vi "Process.vi"(8 "error in":errorcluster, 11 "Inst UI.AH2500":refnum<class "Inst UI.AH2500.lvclass">) -> (0 "error out":errorcluster, 3 "Inst UI.AH2500 out":refnum<class "Inst UI.AH2500.lvclass">)   [LabVIEW 2019, in "Inst UI.AH2500.lvclass"]
doc: "---------------------------------------------------------------\nJKI State Machine Objects™\nhttp://jki.net/state-machine-objects/\nCopyright (C) 2005-2015, JKI <info@jki.net>\nALL RIGHTS RESERVEDJKI State Machine Objects (SMO) 1.0.0.5\nJKI - JKI\nCopyright (c) 2016, JKI"
uses:
  Inst UI.AH2500.lvclass
  C:/Program Files/National Instruments/LabVIEW 2019/vi.lib/JKI/JKI SMO/SMO/SMO.lvclass
  C:/Program Files/National Instruments/LabVIEW 2019/user.lib/LevyLab/Instrument Framework/Instrument UI/Instrument UI.lvclass
  C:/Program Files/National Instruments/LabVIEW 2019/vi.lib/JKI/JKI SMO/SMO.UI/SMO.UI.lvclass
  Inst.AH2500/Typedefs/Inst.AH2500.getAll--Cluster.ctl
  Inst.AH2500/Inst.AH2500.lvclass
  C:/Program Files/National Instruments/LabVIEW 2019/user.lib/LevyLab/Instrument Framework/Instrument/Instrument.lvclass
  Inst UI.AH2500.UI--Cluster.ctl
  Inst.AH2500/Typedefs/Inst.AH2500.Configuration--Cluster.ctl
  <userlib>/LevyLab/Configuration/Configuration.lvclass
  <userlib>/LevyLab/RemoteControl/RemoteControl/Typedefs/Message--Cluster.ctl
  <userlib>/LevyLab/Instrument Framework/Instrument UI/Instrument UI.lvclass/Instrument UI.ctl
  Inst.AH2500/Inst.AH2500.lvclass/Inst.AH2500.ctl
  <vilib>/JKI/JKI SMO/SMO/SMO.lvclass/SMO.ctl
  <userlib>/LevyLab/Configuration/Configuration.lvclass/Configuration.ctl
  <userlib>/LevyLab/Instrument Framework/Instrument/Typedefs/Client Type--Enum.ctl
  <userlib>/LevyLab/Instrument Framework/Instrument/Instrument.lvclass/Instrument.ctl
  f57a6be4-1a14-4c07-88ea-2903807e6527.vi
  <vilib>/JKI/JKI SMO/SMO/Private/ReftoDVR--SMO.vi
  f57a6be4-1a14-4c07-88ea-2903807e6527.vi/3b87bc3d-4873-4b4f-ba08-c078dcd240b2.vi
  f57a6be4-1a14-4c07-88ea-2903807e6527.vi/f27b08c5-9c53-421b-9d46-0768e3ef8b01.vi
  <vilib>/Utility/Data Type/Get Type Information.vi
  <vilib>/JDP Science/JSONtext/JSON text to Variant.vi
  <userlib>/LevyLab/Instrument Framework/Instrument/API/Instrument.sendMessageToProcess (variant).vi
  <userlib>/LevyLab/Instrument Framework/Instrument/Instrument.lvclass
  <vilib>/JDP Science/JSONtext/LVClass Serializer/JSONtext LVClass Serializer.lvclass
  <userlib>/LevyLab/Instrument Framework/Instrument UI/Instrument UI.lvclass
  <vilib>/JKI/JKI SMO/SMO/SMO.lvclass
  <vilib>/JKI/JKI SMO/SMO.UI/SMO.UI.lvclass
  <userlib>/LevyLab/RemoteControl/RemoteControl/RemoteControl.lvclass
  C:/Program Files/National Instruments/LabVIEW 2019/user.lib/LevyLab/Instrument Framework/Instrument Types/CBridge/Instrument.CBridge.lvclass
panel:
  in  "Enable Output 2":bool
  in  "I/O":bool
  out "STUFF":bool
  out "LOSS":string="bridge"
  out "CAPACITANCE - pF":string="cap"
  out "Status":string="SMO State: Stopped"
  out "version":string="vDevelopment"
  # "AH 2500A ULTRA-PRECISION 1kHz CAPACITANCE BRIDGE"
  # "SMO UI Template"
  # "For instructions on how to use the JKI State Machine Objects, examples and video tutorials, visit:\nhttp://jki.net/state-machine-objects/\n\nJKI State Machine Objects™\nhttp://jki.net/state-machine-objects/\nCopyright (C) 2005-2015, JKI <info@jki.net>\nALL RIGHTS RESERVED"
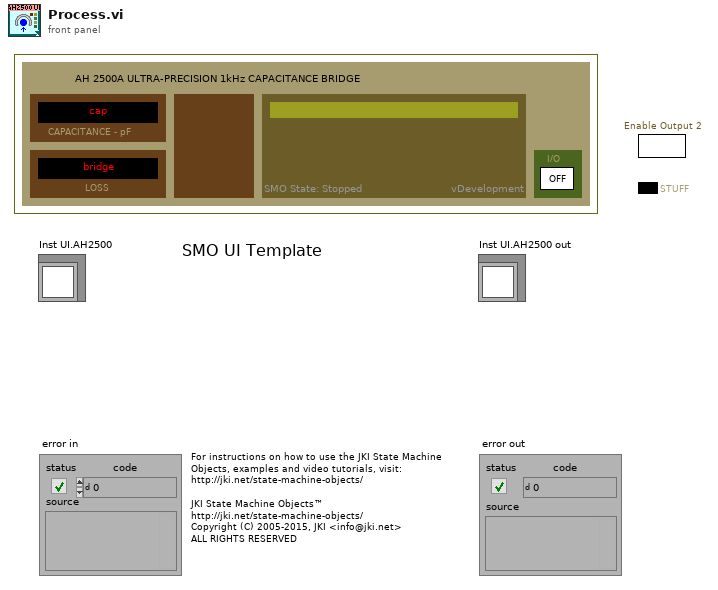
[diagram p1: front panel]
types:
  T1 = enum32{"invalid app kind", "Development System", "Run Time System", "Student Edition", "Embedded LabVIEW", "Evaluation", "Custom"}
  T2 = enum32{"Invalid", "Standard", "Closed", "Hidden", "Minimized", "Maximized"}
  T3 = typedef "Instrument.lvlib/Instrument.lvclass/Client Type--Enum.ctl" = enum16{"Remote", "Local"}
  T4 = typedef "RemoteControl.lvclass/Message--Cluster.ctl" = cluster{"Command":string, "Data":variant, "ID":string}
  T5 = typedef "Inst.AH2500.lvclass/Inst.AH2500.Configuration--Cluster.ctl" = cluster{"Example Setting 1":dbl, "Example Setting 2":dbl, "Example Setting 3":string}
  T6 = typedef "Inst.AH2500.lvclass/Inst.AH2500.getAll--Cluster.ctl" = cluster{"capacitance (pF)":dbl, "loss (nS)":dbl, "Vexc (V)":dbl}
  T7 = typedef "Inst UI.AH2500.lvclass/Inst UI.AH2500.UI--Cluster.ctl" = cluster{"Ch1 (V)":dbl, "Ch2 (V)":dbl, "Slew (V/s)":dbl}
  T8 = typedef "RemoteControl.lvlib/RemoteControl.lvclass/Message--Cluster.ctl" = cluster{"Command":string, "Data":variant, "ID":string}
  T9 = cluster{"Core":cluster{"Current VI Reference":refnum<vi>, "Close Panel on Exit?":bool, "Last Error":cluster{"error":errorcluster, "previous state":string, "remaining states":string}, "Shutdown?":bool}, "Instrument UI":refnum<class "Inst UI.AH2500.lvclass">, "Instrument":refnum<class "Inst.AH2500.lvclass">, "Configuration":refnum<class "Configuration.lvclass">, "Config Cluster":T5, "getAll":T6, "UI Cluster":T7, "Message":T8}
  T10 = cluster{"Current VI Reference":refnum<vi>, "Close Panel on Exit?":bool, "Last Error":cluster{"error":errorcluster, "previous state":string, "remaining states":string}, "Shutdown?":bool}
  T11 = typedef "SMO.lvclass/SMOState --Enum.ctl" = enum16{"unknown", "Created", "Started", "Stopped"}
  T12 = typedef "SMO.lvclass/Protected Events.ctl" = cluster{"StopProcesses":refnum<user-event>, "AbortProcesses":refnum<user-event>, "Config Changed":refnum<user-event>, "Dependency":refnum<user-event>}
  T13 = typedef "Instrument.lvlib/Instrument.lvclass/PublicEvents--Cluster.ctl" = cluster{"MessageFromProcess":refnum<user-event>}
  T14 = typedef "Inst.AH2500.lvclass/PublicEvents--Cluster.ctl" = cluster{"MessageFromProcess":refnum<user-event>}
  T15 = typedef "SMO.lvclass/Public Events.ctl" = cluster{"Error":refnum<user-event>, "State":refnum<user-event>, "Reserve State":refnum<user-event>}
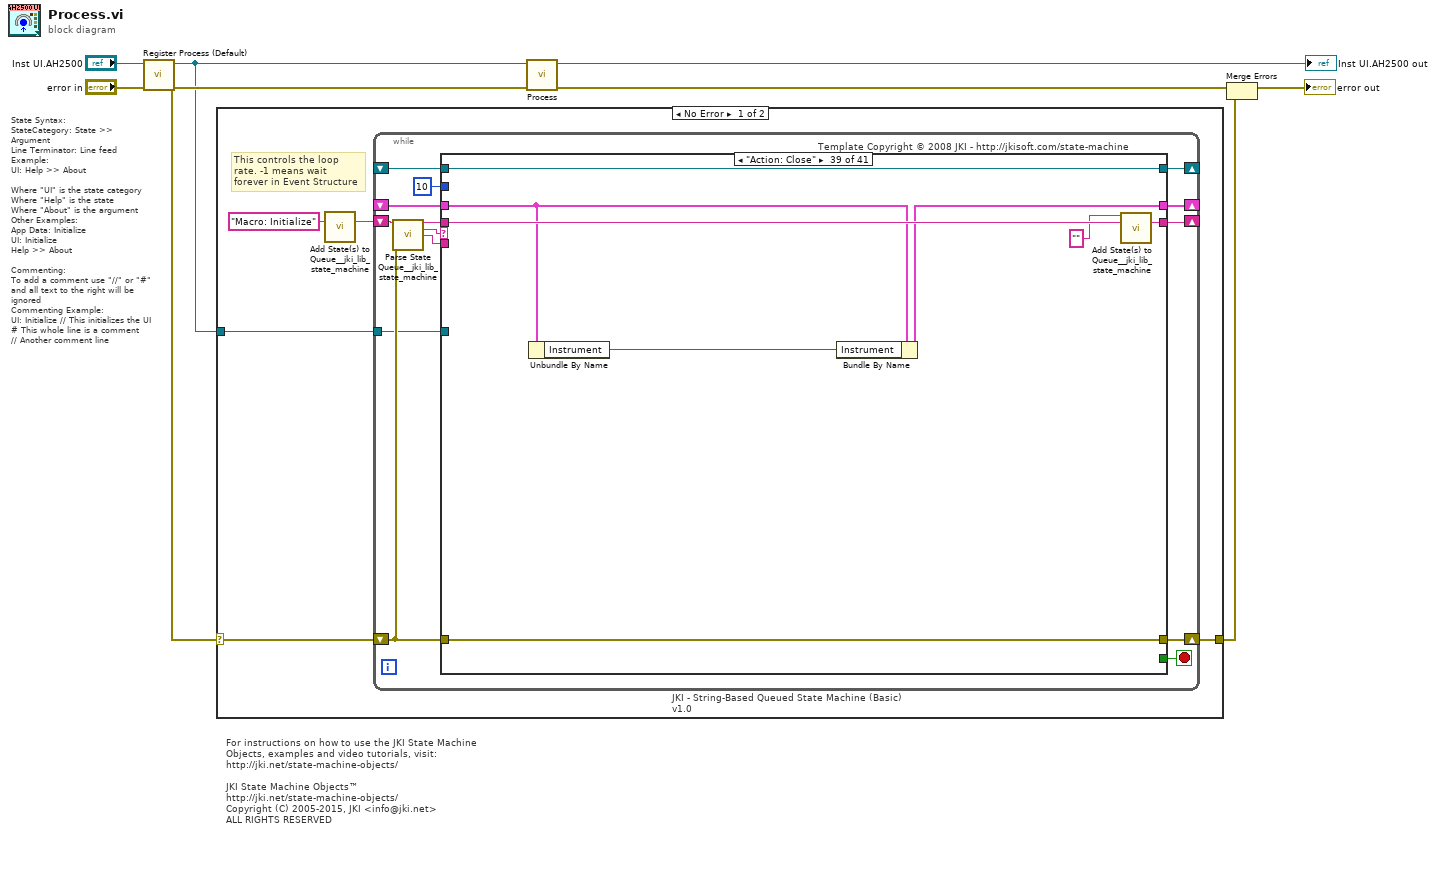
[diagram p0: block diagram]
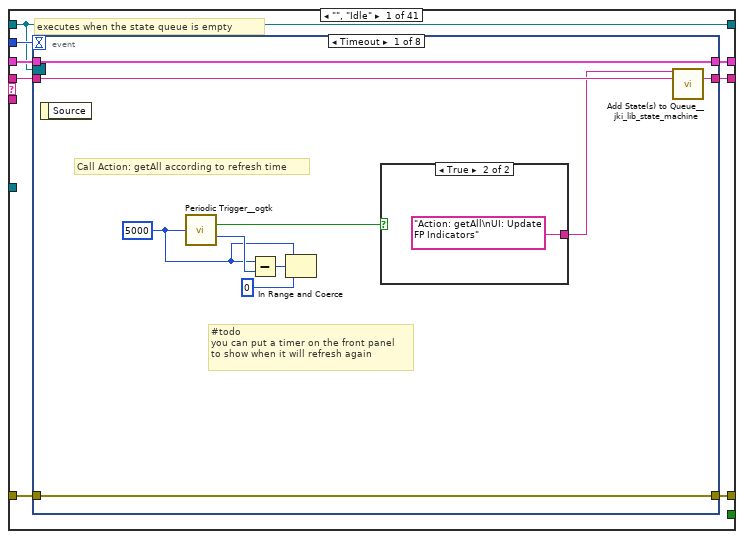
[diagram p2: hidden frame]
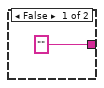
[diagram p3: hidden frame]
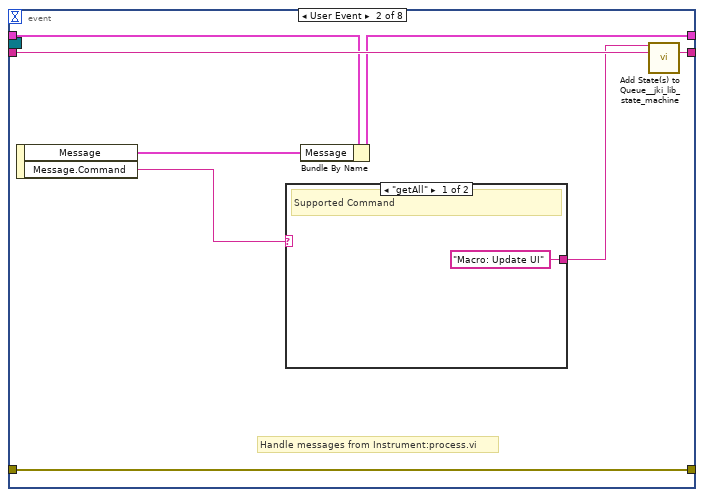
[diagram p4: hidden frame]
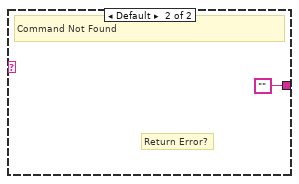
[diagram p5: hidden frame]
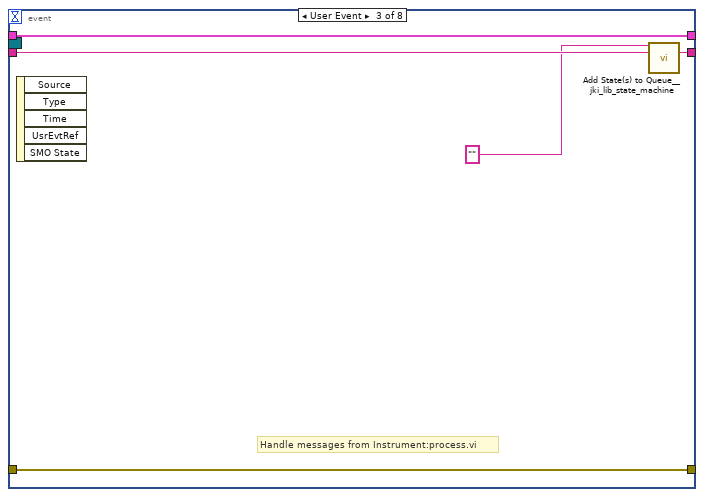
[diagram p6: hidden frame]
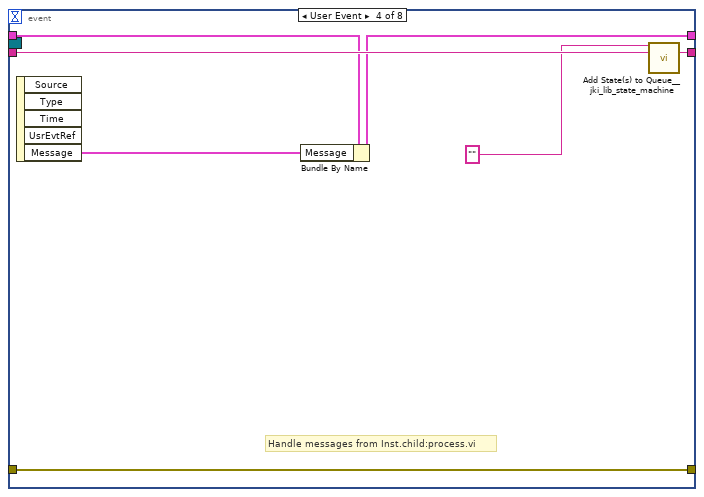
[diagram p7: hidden frame]
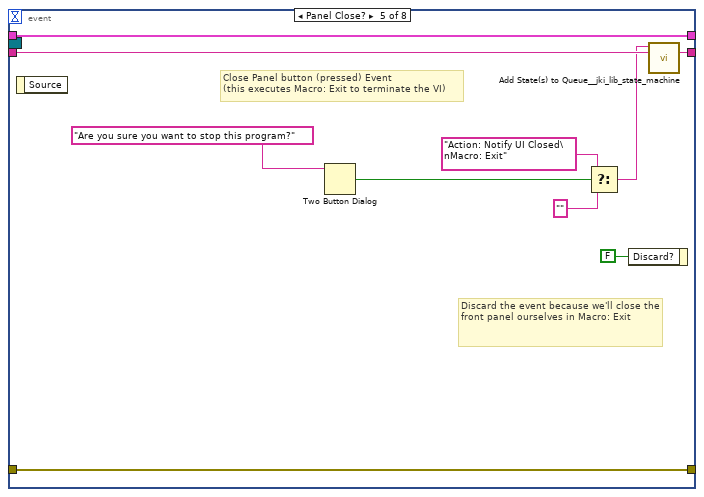
[diagram p8: hidden frame]
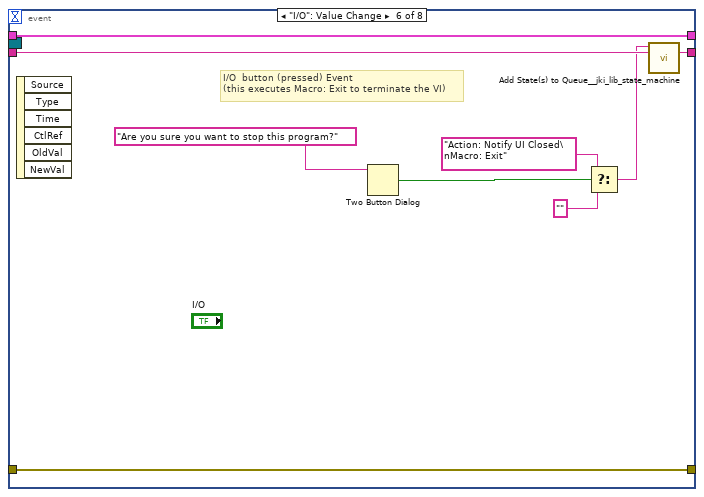
[diagram p9: hidden frame]
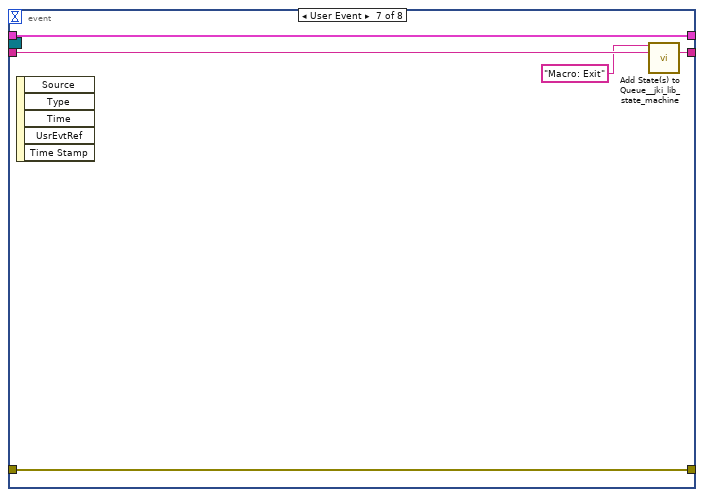
[diagram p10: hidden frame]
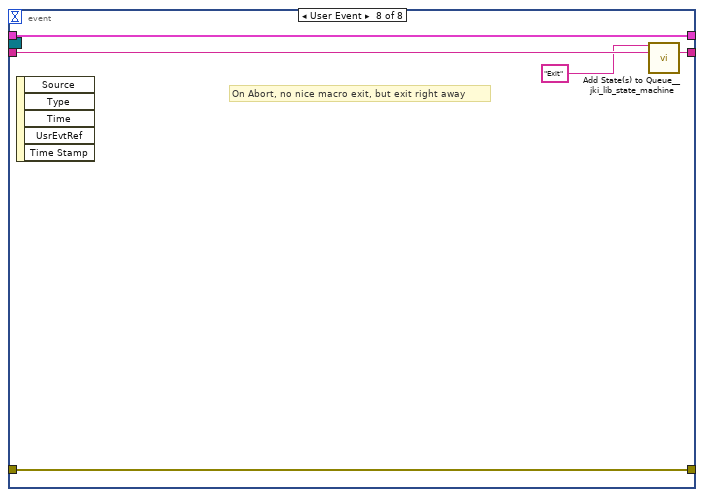
[diagram p11: hidden frame]
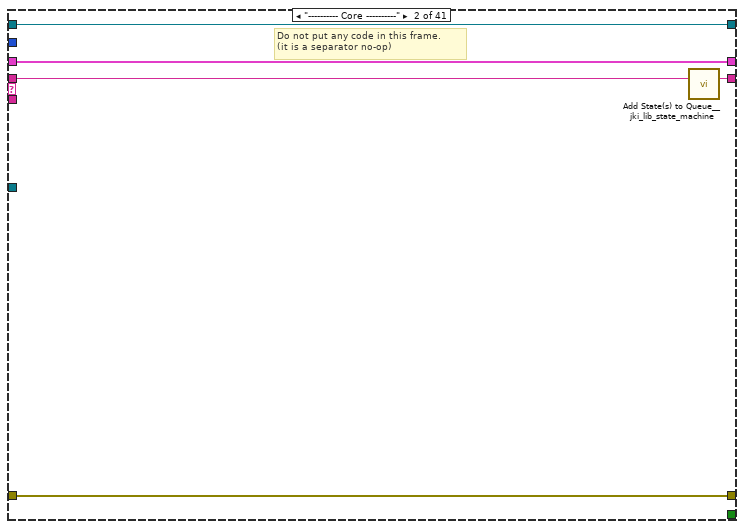
[diagram p12: hidden frame]
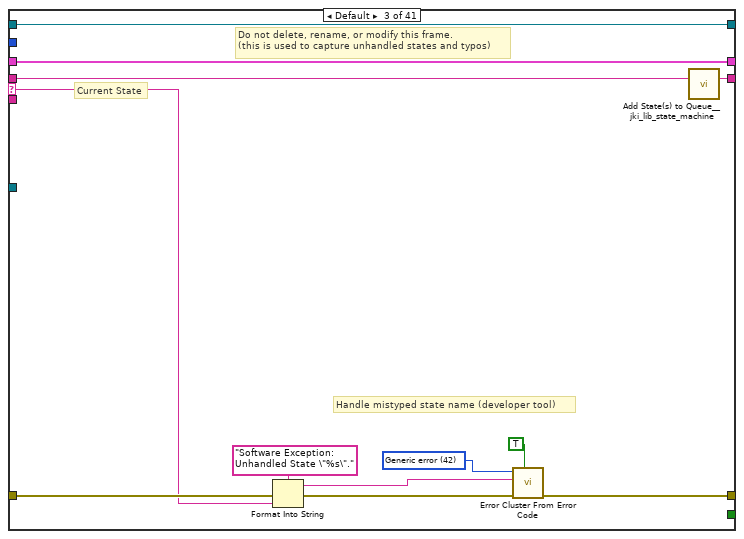
[diagram p13: hidden frame]
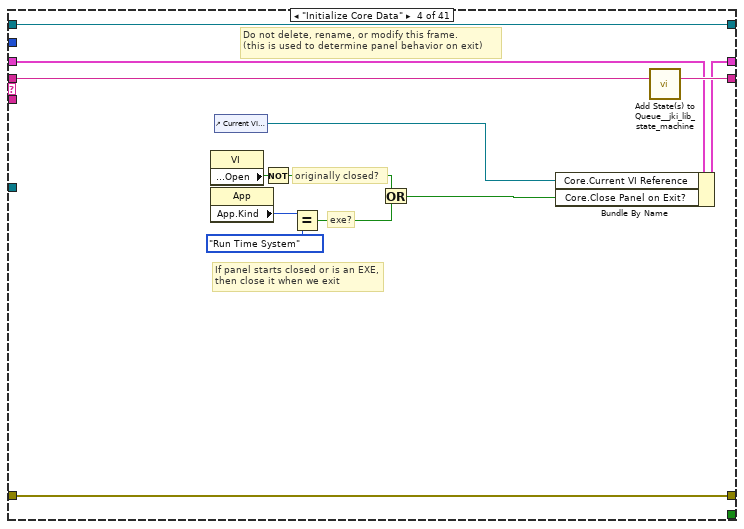
[diagram p14: hidden frame]
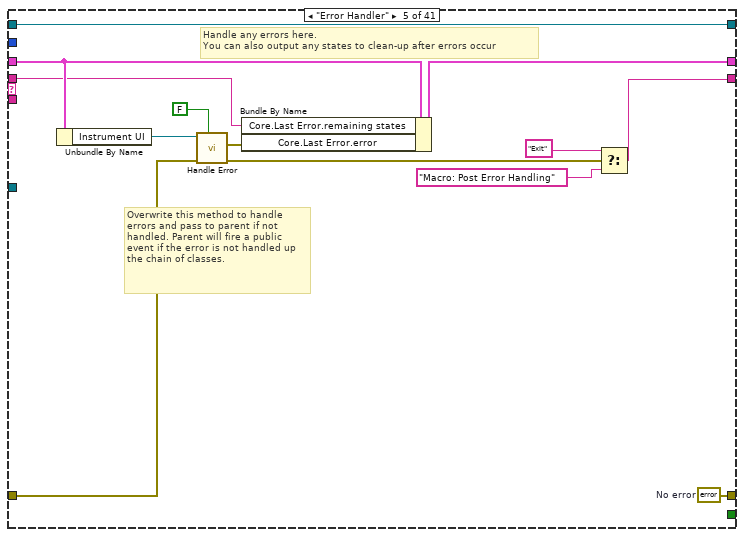
[diagram p15: hidden frame]
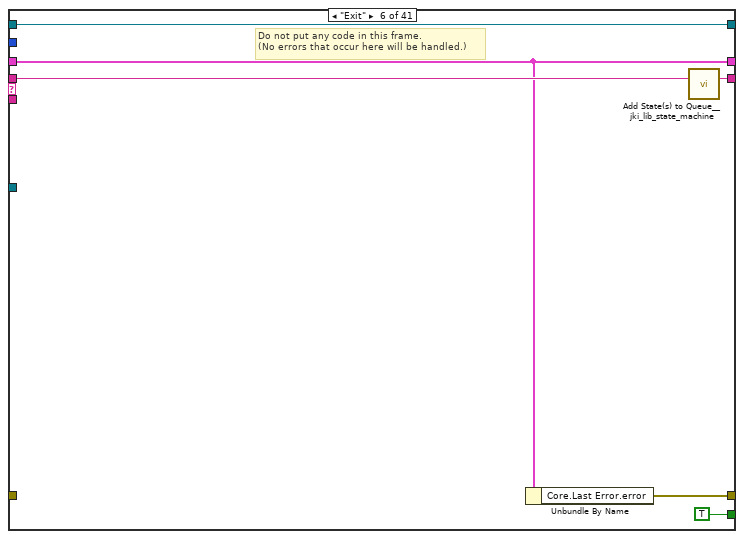
[diagram p16: hidden frame]
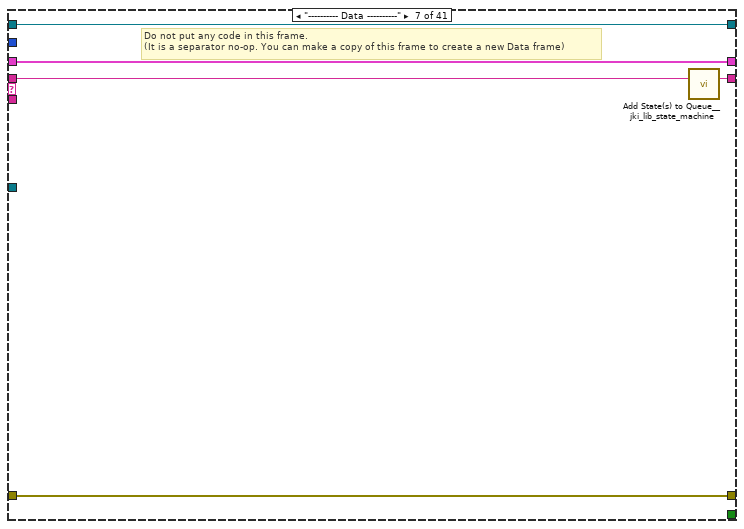
[diagram p17: hidden frame]
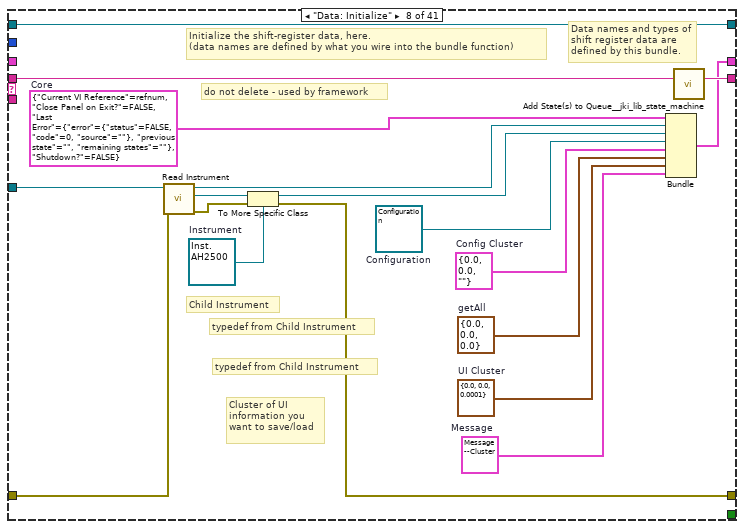
[diagram p18: hidden frame]
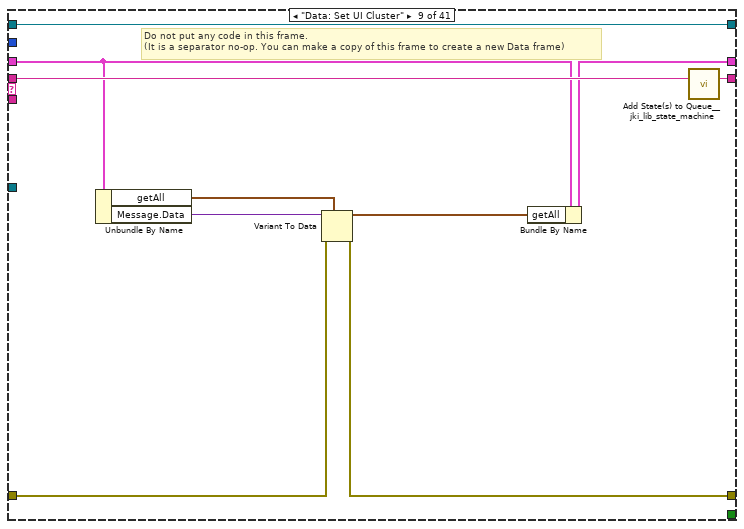
[diagram p19: hidden frame]
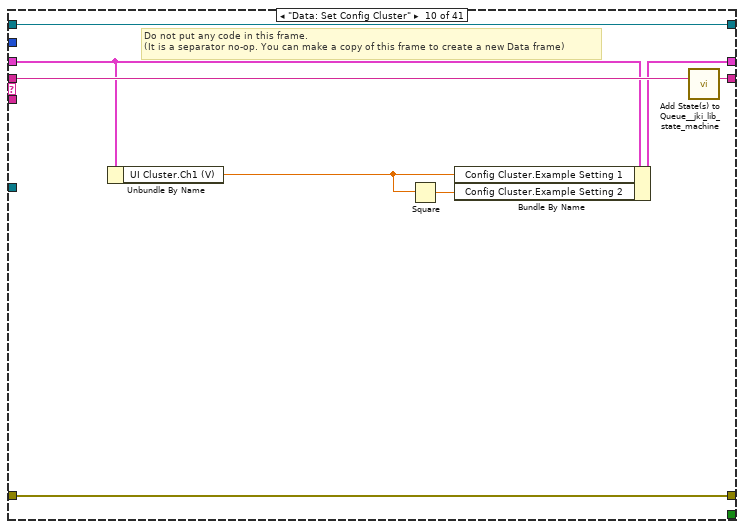
[diagram p20: hidden frame]
diagram:
  # "State Syntax:\nStateCategory: State >> Argument\nLine Terminator: Line feed\nExample:\nUI: Help >> About\n\nWhere \"UI\" is the state category\nWhere \"Help\" is the state\nWhere \"About\" is the argument\nOther Examples:\nApp Data: Initialize\nUI: Initialize\nHelp >> About\n\nCommenting:\nTo add a comment use \"//\" or \"#\" and all text to the right will be ignored\nCommenting Example:\nUI: Initialize // This initializes the UI\n# This whole line is a comment\n// Another comment line"
  # "For instructions on how to use the JKI State Machine Objects, examples and video tutorials, visit:\nhttp://jki.net/state-machine-objects/\n\nJKI State Machine Objects™\nhttp://jki.net/state-machine-objects/\nCopyright (C) 2005-2015, JKI <info@jki.net>\nALL RIGHTS RESERVED"
  n1 = call <vilib>:"Register Process (Default).vi"("error in (no error)"="error in", "SMO"="Inst UI.AH2500") -> ("error out"=w5:errorcluster, "SelfRef"=w4:refnum<class "Inst UI.AH2500.lvclass">)  [unwired: 8 in]
  n2 = case shown="No Error" w5 {
    selector: w5 -> [w10 w509]
    tunnel: w4 -> [w11 _]
    tunnel: [w9 w509] -> w1
    frame No Error {
      # "This controls the loop rate. -1 means wait forever in Event Structure"
      n3 = call <vilib>:"Add State(s) to Queue__jki_lib_state_machine.vi"("State(s) in (\"\")"="Macro: Initialize") -> ("States Out"=w13:string)  [unwired: 14 in]
      n4 = while "JKI - String-Based Queued State Machine (Basic) v1.0" {
        shift-right: [w20] -> _
        shift-left: _ -> [w19]
        shift-right: [w23] -> w9
        shift-left: w10 -> [w17]
        shift-right: [w22] -> _
        shift-left: w13 -> [w24]
        tunnel: w11 -> [w16]
        shift-right: [w15] -> _
        shift-left: _ -> [w14]
        stop <- w21 stop-if-true
        # "Template Copyright © 2008 JKI - http://jkisoft.com/state-machine"
        n5 = call <vilib>:"Parse State Queue__jki_lib_state_machine.vi"("State Queue"=w24, "Error In (no error)"=w17) -> ("Remaining States"=w26:string, "Current State"=w27:string, "Arguments"=w25:string)  [unwired: 11 in]
        n6 = case shown="\"Action: Close\"" w27 {
          selector: w27 -> [_ _ w105 _ _ _ _ _ _ _ _ _ _ _ _ _ _ _ _ _ _ _ _ _ _ _ _ _ _ _ _ _ _ _ _ _ _ _ _ _ _]
          tunnel: w26 -> [w35 w103 w109 w128 w132 w147 w152 w170 w180 w188 w195 w200 w212 w217 w231 w242 w258 w290 w299 w311 w321 w327 w333 w348 w353 w364 w371 w376 w395 w401 w406 w421 w429 w441 w448 w455 w469 w480 w488 w498 w508]
          tunnel: w25 -> [_ _ _ _ _ _ _ _ _ _ _ _ _ _ _ w236 w252 _ _ _ _ _ _ _ _ _ _ _ _ _ _ _ _ _ _ _ _ _ _ _ _]
          tunnel: w19 -> [w33 w100 w107 w119 w135 w143 w149 _ w176 w184 w189 w197 w210 w213 w227 w240 w254 w287 w295 w301 w318 w324 w330 w335 w350 w361 w366 w373 w393 w399 w403 w414 w426 w432 w443 w449 w462 w475 w481 w493 w503]
          tunnel: [w32 w101 w111 w125 w137 w142 w150 w157 w172 w186 w191 w198 w207 w215 w228 w237 w255 w288 w297 w309 w319 w325 w331 w346 w351 w355 w367 w374 w390 w396 w404 w407 w424 w433 w445 w450 w457 w472 w482 w489 w499] -> w23
          tunnel: w17 -> [w31 w101 w110 w125 w131 _ w150 w154 w171 w186 w192 w198 w208 w215 w228 w238 w256 w288 w297 w309 w319 w325 w331 w346 w351 w356 w368 w374 w380 w397 w404 w416 w422 w434 w445 w451 w463 w471 w482 w490 w500]
          tunnel: [w34 w102 w108 w127 w129 w146 w151 w169 w179 w187 w194 w199 w211 w216 w230 w241 w257 w289 w298 w310 w320 w326 w332 w347 w352 w363 w370 w375 w394 w400 w405 w420 w428 w440 w447 w454 w468 w479 w487 w497 w507] -> w22
          tunnel: [_ _ _ _ _ TRUE _ _ _ _ _ _ _ _ _ _ _ _ _ _ _ _ _ _ _ _ _ _ _ _ _ _ _ _ _ _ _ _ _ _ _] -> w21
          tunnel: [w30 w100 w107 w126 w134 w143 w149 w168 w177 w183 w189 w197 w210 w213 w227 w240 w254 w287 w295 w302 w318 w324 w330 w335 w350 w361 w366 w373 w393 w399 w403 w418 w426 w430 w442 w449 w464 w476 w483 w494 w504] -> w20
          tunnel: 10 ("Timeout") -> [w29 _ _ _ _ _ _ _ _ _ _ _ _ _ _ _ _ _ _ _ _ _ _ _ _ _ _ _ _ _ _ _ _ _ _ _ _ _ _ _ _]
          tunnel: w16 -> [_ _ _ _ _ _ _ w155 _ _ _ _ _ _ _ _ _ _ _ _ _ _ _ _ _ _ _ _ _ _ _ _ _ _ _ _ _ _ _ _ _]
          tunnel: [w28 w99 w104 w116 w141 w144 w148 w167 w178 w185 w190 w196 w209 w214 w229 w239 w251 w286 w296 w308 w317 w323 w329 w340 w349 w362 w369 w372 w392 w398 w402 w419 w427 w439 w446 w453 w467 w478 w486 w496 w506] -> w15
          tunnel: w14 -> [w28 w99 w104 w116 w141 w144 w148 w167 w178 w185 w190 w196 w209 w214 w229 w239 w251 w286 w296 w308 w317 w323 w329 w340 w349 w362 w369 w372 _ w398 w402 w419 w427 w439 w446 w453 w467 w478 w486 w496 w506]
          frame "", "Idle" {
            # "executes when the state queue is empty"
            n7 = event shown="[0] Timeout" {
              selector: w28 -> [_ _ _ _ _ _ _ _]
              dyn-events: _ -> [_ _ _ _ _ _ _ _]
              timeout: w29 -> [_ _ _ _ _ _ _ _]
              tunnel: w35 -> [w45 w55 w62 w69 w79 w88 w93 w98]
              tunnel: [w44 w54 w61 w68 w78 w87 w92 w97] -> w34
              tunnel: w33 -> [w42 w52 w58 w66 w76 w86 w90 w95]
              tunnel: [w43 w53 w60 w67 w75 w85 w91 w96] -> w32
              tunnel: w31 -> [w43 w53 w60 w67 w75 w85 w91 w96]
              tunnel: [w42 w51 w58 w65 w76 w86 w90 w95] -> w30
              event Timeout {
                w37 = u32 5000 ("time (ms)")
                # "#todo\nyou can put a timer on the front panel\nto show when it will refresh again"
                # "Call Action: getAll according to refresh time"
                n8 = event-data() -> ()  [unwired: 1 in, 1 out]
                n9 = call <userlib>:"Periodic Trigger__ogtk.vi"("time (ms)"=w37) -> ("Triggered"=w40:bool, "timer value"=w39:u32)  [unwired: 12 in, 1 out]
                n10 = Subtract(x=w37, y=w39) -> (x-y=w38:u32)
                n11 = In Range and Coerce(upper limit=w37, x=w38, lower limit=u32 0) -> ()  [unwired: 2 out]
                n12 = case shown="True" w40 {
                  tunnel: ["" ("State(s) in Front (\"\")") "Action: getAll\nUI: Update FP Indicators" ("State(s) in Front (\"\")")] -> w41
                  frame False {
                  }
                  frame True {
                  }
                }
                n13 = call <vilib>:"Add State(s) to Queue__jki_lib_state_machine.vi"("State(s) in Front (\"\")"=w41, "State(s) in (\"\")"=w45) -> ("States Out"=w44:string)  [unwired: 13 in]
              }
              event User Event {
                # "Handle messages from Instrument:process.vi"
                n14 = event-data() -> ("Message"=w50:T4, "Message.Command"=w48:string)  [unwired: 1 in]
                n15 = case shown="\"getAll\"" w48 {
                  tunnel: ["Macro: Update UI" "" ("Empty String Constant")] -> w49
                  frame "getAll" {
                    # "Supported Command"
                  }
                  frame Default {
                    # "Return Error?"
                    # "Command Not Found"
                  }
                }
                n16 = Bundle By Name(cluster=w52, "Message"=w50) -> (w51:T9)
                n17 = call <vilib>:"Add State(s) to Queue__jki_lib_state_machine.vi"("State(s) in Front (\"\")"=w49, "State(s) in (\"\")"=w55) -> ("States Out"=w54:string)  [unwired: 13 in]
              }
              event User Event {
                # "Handle messages from Instrument:process.vi"
                n18 = event-data() -> ()  [unwired: 1 in, 5 out]
                n19 = call <vilib>:"Add State(s) to Queue__jki_lib_state_machine.vi"("State(s) in Front (\"\")"="" ("State(s) in Front (\"\")"), "State(s) in (\"\")"=w62) -> ("States Out"=w61:string)  [unwired: 13 in]
              }
              event User Event {
                # "Handle messages from Inst.child:process.vi"
                n20 = event-data() -> ("Message"=w63:T4)  [unwired: 1 in, 4 out]
                n21 = Bundle By Name(cluster=w66, "Message"=w63) -> (w65:T9)
                n22 = call <vilib>:"Add State(s) to Queue__jki_lib_state_machine.vi"("State(s) in Front (\"\")"="" ("State(s) in Front (\"\")"), "State(s) in (\"\")"=w69) -> ("States Out"=w68:string)  [unwired: 13 in]
              }
              event Panel Close? {
                # "Discard the event because we'll close the front panel ourselves in Macro: Exit"
                # "Close Panel button (pressed) Event\n(this executes Macro: Exit to terminate the VI)"
                n23 = event-data() -> ()  [unwired: 1 in, 1 out]
                n24 = Two Button Dialog(message="Are you sure you want to stop this program?") -> (T button?=w74:bool)  [unwired: 2 in]
                n25 = Select(t="Action: Notify UI Closed\nMacro: Exit", s=w74, f="") -> (s? t:f=w71:string)
                n26 = event-data("Discard?"=FALSE) -> ()  [unwired: 1 in, 1 out]
                n27 = call <vilib>:"Add State(s) to Queue__jki_lib_state_machine.vi"("State(s) in Front (\"\")"=w71, "State(s) in (\"\")"=w79) -> ("States Out"=w78:string)  [unwired: 13 in]
              }
              event "I/O": Value Change {
                # "I/O  button (pressed) Event\n(this executes Macro: Exit to terminate the VI)"
                n28 = event-data() -> ()  [unwired: 1 in, 6 out]
                n29 = Two Button Dialog(message="Are you sure you want to stop this program?") -> (T button?=w84:bool)  [unwired: 2 in]
                n30 = Select(t="Action: Notify UI Closed\nMacro: Exit", s=w84, f="") -> (s? t:f=w81:string)
                n31 = call <vilib>:"Add State(s) to Queue__jki_lib_state_machine.vi"("State(s) in Front (\"\")"=w81, "State(s) in (\"\")"=w88) -> ("States Out"=w87:string)  [unwired: 13 in]
              }
              event User Event {
                n32 = event-data() -> ()  [unwired: 1 in, 5 out]
                n33 = call <vilib>:"Add State(s) to Queue__jki_lib_state_machine.vi"("State(s) in Front (\"\")"="Macro: Exit", "State(s) in (\"\")"=w93) -> ("States Out"=w92:string)  [unwired: 13 in]
              }
              event User Event {
                # "On Abort, no nice macro exit, but exit right away"
                n34 = event-data() -> ()  [unwired: 1 in, 5 out]
                n35 = call <vilib>:"Add State(s) to Queue__jki_lib_state_machine.vi"("State(s) in Front (\"\")"="Exit", "State(s) in (\"\")"=w98) -> ("States Out"=w97:string)  [unwired: 13 in]
              }
            }
          }
          frame "---------- Core ----------" {
            # "Do not put any code in this frame.\n(it is a separator no-op)"
            n36 = call <vilib>:"Add State(s) to Queue__jki_lib_state_machine.vi"("State(s) in (\"\")"=w103) -> ("States Out"=w102:string)  [unwired: 14 in]
          }
          frame Default {
            w114 = 42 items=["No error", "Argument error", "Memory is full", "Out of zone", "End of file", "File already open", "Generic file I/O error", "File not found", "File permission error", "Disk is full", "Duplicate path", "Too many files open", "System feature not enabled", "Resource file not found", "Cannot add resource", "Resource not found", "Image not found", "Image memory error", "Pen does not exist", "Config type invalid", "Config token not found", "Config parse error", "Config memory error", "Bad external code format", "Bad external code offset", "External code not present", "Null window", "Destroy window error", "Null menu", "Print aborted", "Bad print record", "Print driver error", "Windows error during printing", "Memory error during printing", "Print dialog error", "Generic print error", "Invalid device refnum", "Device not found", "Device parameter error", "Device unit error", "Cannot open device", "Device call aborted", "Generic error", "Cancelled by user", "Object ID too low", "Object ID too high", "Object not in heap", "Unknown heap", "Unknown object (invalid DefProc)", "Unknown object (DefProc not in table)", "Message out of range", "Invalid (null) method", "Unknown message", "Manager call not supported", "Bad address", "Network operation in progress", "Network operation timed out", "Connection is busy", "Network attribute not supported", "Network error", "Address in use", "System out of memory", "Connection aborted", "Connection refused", "Not connected", "Already connected", "Connection closed", "Initialization error (interapplication manager)", "Bad occurrence", "Wait on unbound occurrence handler", "Occurrence queue overflow", "Datalog type conflict", "Unused", "Unrecognized type (interapplication manager)", "Memory corrupt", "Failed to make temporary DLL", "Old CIN version", "Drag socket not found", "Failed to load drop-object", "Failed to register OLE object", "Failed to release OLE object", "Format specifier type mismatch", "Unknown format specifier", "Too few format specifiers", "Too many format specifiers", "Scan failed", "Newer CIN version", "Error converting to variant", "Runtime menu error", "Password tampered", "Variant attribute not found", "Incompatible variant data type", "Event data is not available", "Event Store is not present", "Occurrence is not found", "Event Queue is not created", "Event info is not available", "Refnum passed is NULL", "Error retrieving Class GUID", "Error retrieving CoClass GUID", "Error retrieving TypeLib GUID.", "Bad built application magic bytes.", "Specific driver is different from the specific driver associated with the Logical Name.", "There is no session opened to the class driver.", "Max Error", "MAX - Error with config objects", "MAX - Error loading configuration", "MAX - Group not supported"]
            # "Current State"
            # "Do not delete, rename, or modify this frame.\n(this is used to capture unhandled states and typos)"
            # "Handle mistyped state name (developer tool)"
            n37 = Format Into String(format string="Software Exception: Unhandled State \"%s\"." ("message"), error in=w110, w105) -> (resulting string=w113:string, error out=w112:errorcluster)  [unwired: 1 in]
            n38 = call <vilib>:"Error Cluster From Error Code.vi"("show call chain? (False)"=TRUE, "error in (no error)"=w112, "error message (\"\")"=w113, "error code (0)"=w114) -> ("error out"=w111:errorcluster)  [unwired: 5 in]
            n39 = call <vilib>:"Add State(s) to Queue__jki_lib_state_machine.vi"("State(s) in (\"\")"=w109) -> ("States Out"=w108:string)  [unwired: 14 in]
          }
          frame "Initialize Core Data" {
            # "Do not delete, rename, or modify this frame.\n(this is used to determine panel behavior on exit)"
            # "originally closed?"
            # "exe?"
            # "If panel starts closed or is an EXE, then close it when we exit"
            n40 = property class="VI"() -> ("Front Panel.Open"=w124:bool)  [unwired: 2 in, 2 out]
            n41 = property class="App"() -> ("App.Kind"=w123:T1)  [unwired: 2 in, 2 out]
            n42 = control-ref of="Current VI Reference"() -> (w117:refnum<vi>)
            n43 = Not(x=w124) -> (.not. x?=w121:bool)
            n44 = Equal?(x=w123, y=T1."Run Time System" ("Application:Kind")) -> (x = y?=w120:bool)
            n45 = Or(x=w121, y=w120) -> (x .or. y?=w118:bool)
            n46 = Bundle By Name(cluster=w119, "Core.Current VI Reference"=w117, "Core.Close Panel on Exit?"=w118) -> (w126:T9)
            n47 = call <vilib>:"Add State(s) to Queue__jki_lib_state_machine.vi"("State(s) in (\"\")"=w128) -> ("States Out"=w127:string)  [unwired: 14 in]
          }
          frame "Error Handler" {
            w137 = errorcluster {"status"=FALSE, "code"=0, "source"=""}  # No error
            # "Overwrite this method to handle errors and pass to parent if not handled. Parent will fire a public event if the error is not handled up the chain of classes."
            # "Handle any errors here.\nYou can also output any states to clean-up after errors occur"
            n48 = Unbundle By Name(w135) -> ("Instrument UI"=w140:refnum<class "Inst UI.AH2500.lvclass">)
            n49 = call-dynamic "Handle Error.vi"("Stop on Unhandled Error (T)"=FALSE, "error in"=w131, "SMO"=w140) -> ("handling error"=w138:errorcluster, "Unhandled error"=w136:errorcluster)  [unwired: 6 in, 1 out]
            n50 = Bundle By Name(cluster=w135, "Core.Last Error.remaining states"=w132, "Core.Last Error.error"=w136) -> (w134:T9)
            n51 = Select(t="Exit", s=w138, f="Macro: Post Error Handling") -> (s? t:f=w129:string)
          }
          frame "Exit" {
            # "Do not put any code in this frame.\n(No errors that occur here will be handled.)"
            n52 = Unbundle By Name(w143) -> ("Core.Last Error.error"=w142:errorcluster)
            n53 = call <vilib>:"Add State(s) to Queue__jki_lib_state_machine.vi"("State(s) in (\"\")"=w147) -> ("States Out"=w146:string)  [unwired: 14 in]
          }
          frame "---------- Data ----------" {
            # "Do not put any code in this frame.\n(It is a separator no-op. You can make a copy of this frame to create a new Data frame)"
            n54 = call <vilib>:"Add State(s) to Queue__jki_lib_state_machine.vi"("State(s) in (\"\")"=w152) -> ("States Out"=w151:string)  [unwired: 14 in]
          }
          frame "Data: Initialize" {
            w153 = T8 {"Command"="", "Data"=variant, "ID"=""}  # Message
            w156 = refnum<class "Configuration.lvclass"> refnum  # Configuration
            w159 = T5 {"Example Setting 1"=0.0, "Example Setting 2"=0.0, "Example Setting 3"=""}  # Config Cluster
            w161 = T7 {"Ch1 (V)"=0.0, "Ch2 (V)"=0.0, "Slew (V/s)"=0.0001}  # UI Cluster
            w163 = refnum<class "Inst.AH2500.lvclass"> refnum  # Instrument
            w165 = T6 {"capacitance (pF)"=0.0, "loss (nS)"=0.0, "Vexc (V)"=0.0}  # getAll
            w166 = T10 {"Current VI Reference"=refnum, "Close Panel on Exit?"=FALSE, "Last Error"={"error"={"status"=FALSE, "code"=0, "source"=""}, "previous state"="", "remaining states"=""}, "Shutdown?"=FALSE}  # Core
            # "typedef from Child Instrument"
            # "Cluster of UI\ninformation you\nwant to save/load"
            # "Child Instrument"
            # "typedef from Child Instrument"
            # "do not delete - used by framework"
            # "Data names and types of shift register data are defined by this bundle."
            # "Initialize the shift-register data, here.\n(data names are defined by what you wire into the bundle function)"
            n55 = call <userlib>:"Read Instrument.vi"("error in (no error)"=w154, "Instrument UI in"=w155) -> ("error out"=w160:errorcluster, "Instrument"=w162:refnum<class "Instrument.lvclass">, "Instrument UI"=w164:refnum<class "Inst UI.AH2500.lvclass">)  [unwired: 7 in]
            n56 = To More Specific Class(target class=w163, reference=w162, error in=w160) -> (specific class reference=w158:refnum<class "Inst.AH2500.lvclass">, error out=w157:errorcluster)
            n57 = Bundle("Core"=w166, "Instrument UI"=w164, "Instrument"=w158, "Configuration"=w156, "Config Cluster"=w159, "getAll"=w165, "UI Cluster"=w161, "Message"=w153) -> (w168:T9)  [unwired: 1 in]
            n58 = call <vilib>:"Add State(s) to Queue__jki_lib_state_machine.vi"("State(s) in (\"\")"=w170) -> ("States Out"=w169:string)  [unwired: 14 in]
          }
          frame "Data: Set UI Cluster" {
            # "Do not put any code in this frame.\n(It is a separator no-op. You can make a copy of this frame to create a new Data frame)"
            n59 = Unbundle By Name(w176) -> ("getAll"=w175:T6, "Message.Data"=w174:variant)
            n60 = Variant To Data(error in=w171, type=w175, Variant=w174) -> (data=w173:T6, error out=w172:errorcluster)
            n61 = Bundle By Name(cluster=w176, "getAll"=w173) -> (w177:T9)
            n62 = call <vilib>:"Add State(s) to Queue__jki_lib_state_machine.vi"("State(s) in (\"\")"=w180) -> ("States Out"=w179:string)  [unwired: 14 in]
          }
          frame "Data: Set Config Cluster" {
            # "Do not put any code in this frame.\n(It is a separator no-op. You can make a copy of this frame to create a new Data frame)"
            n63 = Unbundle By Name(w184) -> ("UI Cluster.Ch1 (V)"=w182:dbl)
            n64 = Square(x=w182) -> (x^2=w181:dbl)
            n65 = Bundle By Name(cluster=w184, "Config Cluster.Example Setting 1"=w182, "Config Cluster.Example Setting 2"=w181) -> (w183:T9)
            n66 = call <vilib>:"Add State(s) to Queue__jki_lib_state_machine.vi"("State(s) in (\"\")"=w188) -> ("States Out"=w187:string)  [unwired: 14 in]
          }
          frame "Data: Cleanup" {
            # "Cleanup any data and references, here.\n(this is called automatically, by the Macro: Exit)"
            n67 = Unbundle By Name(w189) -> ("Core.Current VI Reference"=w193:refnum<vi>)
            n68 = Close Reference(reference=w193, error in (no error)=w192) -> (error out=w191:errorcluster)
            n69 = call <vilib>:"Add State(s) to Queue__jki_lib_state_machine.vi"("State(s) in (\"\")"=w195) -> ("States Out"=w194:string)  [unwired: 14 in]
          }
          frame "---------- UI ----------" {
            # "Do not put any code in this frame.\n(It is a separator no-op. You can make a copy of this frame to create a new UI frame)"
            n70 = call <vilib>:"Add State(s) to Queue__jki_lib_state_machine.vi"("State(s) in (\"\")"=w200) -> ("States Out"=w199:string)  [unwired: 14 in]
          }
          frame "UI: Initialize" {
            # "size window to decoration box on front panel"
            # "Initialize the User Interface, here.\n(this is called automatically, by the Macro: Init)"
            n71 = call <userlib>:"MGI Get Executable Version.vi"() -> ("Version"=w205:string)  [unwired: 7 in]
            n72 = Format Into String(format string="v%s", w205) -> (resulting string=→"version":string)  [unwired: 2 in, 1 out]
            n73 = call <userlib>:"Fit VI window to Largest Dec__ogtk.vi"("error in (no error)"=w208, "border spacing (2 px)"=0) -> ("error out"=w207:errorcluster)  [unwired: 4 in, 1 out]
            n74 = local write "LOSS"("C bridge" ("LOSS")) -> ()
            n75 = local write "CAPACITANCE - pF"("AH 2500" ("CAPACITANCE - pF")) -> ()
            n76 = call <vilib>:"Add State(s) to Queue__jki_lib_state_machine.vi"("State(s) in (\"\")"=w212) -> ("States Out"=w211:string)  [unwired: 14 in]
          }
          frame "UI: Update FP Controls" {
            # "Do not put any code in this frame.\n(It is a separator no-op. You can make a copy of this frame to create a new UI frame)"
            n77 = Unbundle By Name(w213) -> ()  [unwired: 3 out]
            n78 = call <vilib>:"Add State(s) to Queue__jki_lib_state_machine.vi"("State(s) in (\"\")"=w217) -> ("States Out"=w216:string)  [unwired: 14 in]
          }
          frame "UI: Update FP Indicators" {
            n79 = Unbundle By Name(w227) -> ("getAll"=w226:T6, "Instrument"=w219:refnum<class "Inst.AH2500.lvclass">)
            n80 = First Call?() -> (First Call?: T/F=w218:bool)
            n81 = Unbundle By Name(w226) -> ("capacitance (pF)"=w221:dbl, "loss (nS)"=w220:dbl)  [unwired: 1 out]
            n82 = case shown="True" w218 {
              tunnel: w219 -> [_ w235]
              frame False {
              }
              frame True {
                n83 = call <vilib>:"GetState.vi"("SMO"=w235) -> ("SMO State"=w232:T11)  [unwired: 8 in, 2 out]
                n84 = Format Into String(format string="SMO State: %s", w232) -> (resulting string=→"Status":string)  [unwired: 2 in, 1 out]
              }
            }
            n85 = Format Into String(format string="%08.7f" ("Status 6"), w220) -> (resulting string=→"LOSS":string)  [unwired: 2 in, 1 out]
            n86 = Format Into String(format string="%08.7f" ("Status 6"), w221) -> (resulting string=→"CAPACITANCE - pF":string)  [unwired: 2 in, 1 out]
            n87 = call <vilib>:"Add State(s) to Queue__jki_lib_state_machine.vi"("State(s) in (\"\")"=w231) -> ("States Out"=w230:string)  [unwired: 14 in]
          }
          frame "UI: Cursor Set" {
            # "Argument"
            # "Initialize the User Interface, here.\n(this is called automatically, by the Macro: Init)"
            n88 = disable-structure shown="Default" {
              disable-tunnel: w238 -> [w243 w246]
              disable-tunnel: [w243 w245] -> w237
              disable-tunnel: w236 -> [_ w244]
              frame condition #0 {
              }
              frame condition #1 (active) {
                n89 = case shown="\"Busy\"" w244 {
                  tunnel: w246 -> [w248 w250]
                  tunnel: [w247 w249] -> w245
                  frame "Idle", Default {
                    n90 = call <vilib>:"Unset Busy.vi"("error in (no error)"=w248) -> ("error out"=w247:errorcluster)  [unwired: 10 in]
                  }
                  frame "Busy" {
                    n91 = call <vilib>:"Set Busy.vi"("error in (no error)"=w250) -> ("error out"=w249:errorcluster)  [unwired: 9 in, 1 out]
                  }
                }
              }
            }
            n92 = call <vilib>:"Add State(s) to Queue__jki_lib_state_machine.vi"("State(s) in (\"\")"=w242) -> ("States Out"=w241:string)  [unwired: 14 in]
          }
          frame "UI: Front Panel State" {
            # "Argument"
            # "Set Front Panel Open or Closed\n(Usage: \"UI: Front Panel State >> Open|Close\")"
            n93 = Unbundle By Name(w254) -> ("Core.Current VI Reference"=w253:refnum<vi>)
            n94 = disable-structure shown="Default" {
              disable-tunnel: w256 -> [w262 w285]
              disable-tunnel: [w261 w285] -> w255
              disable-tunnel: w253 -> [w260 _]
              disable-tunnel: w252 -> [w259 _]
              frame condition #0 (active) {
                n95 = case shown="\"Close\"" w259 {
                  tunnel: w262 -> [w266 w279]
                  tunnel: [w268 w280] -> w261
                  tunnel: w260 -> [w267 w277]
                  frame "Open", Default {
                    n96 = property class="VI"(reference=w267, error in=w266) -> (reference out=w264:refnum<vi>, error out=w265:errorcluster, "FP.State"=w263:T2)
                    n97 = case shown="\"Closed\"" w263 {
                      tunnel: [w271 w274] -> w268
                      tunnel: w265 -> [w270 w274]
                      tunnel: w264 -> [w269 _]
                      frame "Closed" {
                        n98 = invoke class="VI" method="FP.Open"(reference=w269, error in=w270, "Activate"=TRUE, "State"=T2."Standard") -> (error out=w271:errorcluster)  [unwired: 1 in, 4 out]
                      }
                      frame Default {
                      }
                    }
                  }
                  frame "Close" {
                    n99 = property class="VI"(reference=w277, error in=w279) -> (reference out=w276:refnum<vi>, error out=w278:errorcluster, "FP.State"=w275:T2)
                    n100 = case shown="Default" w275 {
                      tunnel: [w281 w284] -> w280
                      tunnel: w278 -> [w281 w283]
                      tunnel: w276 -> [_ w282]
                      frame "Invalid", "Closed" {
                      }
                      frame Default {
                        n101 = invoke class="VI" method="FP.Close"(reference=w282, error in=w283) -> (error out=w284:errorcluster)  [unwired: 1 in, 2 out]
                      }
                    }
                  }
                }
              }
              frame condition #1 {
              }
            }
            n102 = call <vilib>:"Add State(s) to Queue__jki_lib_state_machine.vi"("State(s) in (\"\")"=w258) -> ("States Out"=w257:string)  [unwired: 14 in]
          }
          frame "---------- Macro ----------" {
            # "Do not put any code in this frame.\n(It is a separator no-op. You can make a copy of this frame to create a new Macro frame)"
            n103 = call <vilib>:"Add State(s) to Queue__jki_lib_state_machine.vi"("State(s) in (\"\")"=w290) -> ("States Out"=w289:string)  [unwired: 14 in]
          }
          frame "Macro: Initialize" {
            w293 = "UI: Initialize\nMacro: Read UI Config\nAction: Open\n//UI: Front Panel State >> Open\nAction: getAll\nUI: Update FP Indicators"  # UI: Initialize Macro: Read UI Config Action: Open //UI: Front Panel State >> Open Action: getAll UI: Update FP Indicators
            # "Initialization Macro\n(This is called once, when the VI starts)"
            n104 = call <vilib>:"Add State(s) to Queue__jki_lib_state_machine.vi"("State(s) in Front (\"\")"="Data: Initialize\nInitialize Core Data\nEvents: Register", "State(s) in (\"\")"="Process: Sync", "State(s) at Back (\"\")"=w293) -> ("States Out"=w292:string)  [unwired: 12 in]
            n105 = call <vilib>:"Add State(s) to Queue__jki_lib_state_machine.vi"("State(s) in Front (\"\")"=w292, "State(s) in (\"\")"=w299) -> ("States Out"=w298:string)  [unwired: 13 in]
          }
          frame "Macro: Post Error Handling" {
            # "Clear Last Error?"
            n106 = Unbundle By Name(w301) -> ("Core.Last Error.remaining states"=w303:string, "Core.Shutdown?"=w304:bool)
            n107 = Unbundle By Name(w301) -> ("Core.Last Error.error"=w307:errorcluster)
            n108 = case shown="False" FALSE {
              tunnel: w307 -> [w315 _]
              tunnel: [w315 _] -> w306
              frame False {
              }
              frame True {
              }
            }
            n109 = case shown="False" w304 {
              tunnel: w303 -> [w312 w314]
              tunnel: [w312 w313] -> w300
              frame False {
                # "These are the remaining states (at the moment the error occured). States can be altered according to business logic."
                # "NOT SHUTTING DOWN"
              }
              frame True {
                # "Developer can decide to alter the states but should be aware that during the shutdown process, there are certain states that must be run for the SMO to properly shut itself (and this process) down. As such, one can add states to perform additional clean-ups, but should append the remaining state to be executed."
                # "SHUTTING DOWN"
                n110 = call <vilib>:"Add State(s) to Queue__jki_lib_state_machine.vi"("State(s) in (\"\")"=w314) -> ("States Out"=w313:string)  [unwired: 14 in]
              }
            }
            n111 = Bundle By Name(cluster=w301, "Core.Last Error.error"=w306) -> (w302:T9)
            n112 = call <vilib>:"Add State(s) to Queue__jki_lib_state_machine.vi"("State(s) in Front (\"\")"=w300, "State(s) in (\"\")"=w311) -> ("States Out"=w310:string)  [unwired: 13 in]
          }
          frame "Macro: Update UI" {
            # "Do not put any code in this frame.\n(It is a separator no-op. You can make a copy of this frame to create a new Macro frame)"
            n113 = call <vilib>:"Add State(s) to Queue__jki_lib_state_machine.vi"("State(s) in Front (\"\")"="Data: Set UI Cluster\nUI: Update FP Controls" ("State(s) in Front (\"\")"), "State(s) in (\"\")"=w321) -> ("States Out"=w320:string)  [unwired: 13 in]
          }
          frame "Macro: Read UI Config" {
            # "Do not put any code in this frame.\n(It is a separator no-op. You can make a copy of this frame to create a new Macro frame)"
            n114 = call <vilib>:"Add State(s) to Queue__jki_lib_state_machine.vi"("State(s) in Front (\"\")"="Configuration: Initialize\nConfiguration: Read UI Config File\nUI: Update FP Controls" ("State(s) in Front (\"\")"), "State(s) in (\"\")"=w327) -> ("States Out"=w326:string)  [unwired: 13 in]
          }
          frame "Macro: Write UI Config" {
            # "Do not put any code in this frame.\n(It is a separator no-op. You can make a copy of this frame to create a new Macro frame)"
            n115 = call <vilib>:"Add State(s) to Queue__jki_lib_state_machine.vi"("State(s) in Front (\"\")"="Data: Set UI Cluster\nConfiguration: Write UI Config File" ("State(s) in Front (\"\")"), "State(s) in (\"\")"=w333) -> ("States Out"=w332:string)  [unwired: 13 in]
          }
          frame "Macro: Exit" {
            # "Exit Macro\n(This is called once, when the VI exits)"
            n116 = Unbundle By Name(w335) -> ("Core.Close Panel on Exit?"=w345:bool)
            n117 = Select(t="UI: Front Panel State >> Close", s=w345, f="" ("Empty String Constant")) -> (s? t:f=w342:string)
            n118 = call <vilib>:"Add State(s) to Queue__jki_lib_state_machine.vi"("State(s) in Front (\"\")"="Data: Cleanup\nEvents: Unregister\nProcess: Self Terminate", "State(s) in (\"\")"="Process: Sync", "State(s) at Back (\"\")"="Exit") -> ("States Out"=w337:string)  [unwired: 12 in]
            n119 = call <vilib>:"Add State(s) to Queue__jki_lib_state_machine.vi"("State(s) in Front (\"\")"="Action: Close\nMacro: Write UI Config", "State(s) in (\"\")"=w342, "State(s) at Back (\"\")"=w337) -> ("States Out"=w341:string)  [unwired: 12 in]
            n120 = call <vilib>:"Add State(s) to Queue__jki_lib_state_machine.vi"("State(s) in Front (\"\")"=w341, "State(s) in (\"\")"=w348) -> ("States Out"=w347:string)  [unwired: 13 in]
          }
          frame "---------- Process ----------" {
            # "Template Separator\n(You can make a copy of, or modify, this frame)"
            n121 = call <vilib>:"Add State(s) to Queue__jki_lib_state_machine.vi"("State(s) in (\"\")"=w353) -> ("States Out"=w352:string)  [unwired: 14 in]
          }
          frame "Process: Sync" {
            n122 = Unbundle By Name(w361) -> ("Instrument UI"=w357:refnum<class "Inst UI.AH2500.lvclass">)
            n123 = call <vilib>:"WaitOnProcessSync.vi"("error in (no error)"=w356, "SMO"=w357) -> ("error out"=w355:errorcluster, "Don't run?"=w360:bool)  [unwired: 7 in, 1 out]
            n124 = Select(t="Data: Cleanup\nEvents: Unregister\nExit", s=w360, f="" ("Empty String Constant")) -> (s? t:f=w354:string)
            n125 = call <vilib>:"Add State(s) to Queue__jki_lib_state_machine.vi"("State(s) in Front (\"\")"=w354, "State(s) in (\"\")"=w364) -> ("States Out"=w363:string)  [unwired: 13 in]
          }
          frame "Process: Self Terminate" {
            n126 = Unbundle By Name(w366) -> ("Instrument UI"=w365:refnum<class "Inst UI.AH2500.lvclass">)
            n127 = call <vilib>:"SelfTerminate.vi"("error in (no error)"=w368, "SMO in"=w365) -> ("error out"=w367:errorcluster)  [unwired: 8 in, 1 out]
            n128 = call <vilib>:"Add State(s) to Queue__jki_lib_state_machine.vi"("State(s) in (\"\")"=w371) -> ("States Out"=w370:string)  [unwired: 14 in]
          }
          frame "---------- Events ----------" {
            # "Template Separator\n(You can make a copy of, or modify, this frame)"
            n129 = call <vilib>:"Add State(s) to Queue__jki_lib_state_machine.vi"("State(s) in (\"\")"=w376) -> ("States Out"=w375:string)  [unwired: 14 in]
          }
          frame "Events: Register" {
            # "Expand to add\nmore events"
            # "Base Class Protected Events"
            n130 = Unbundle By Name(w393) -> ("Instrument UI"=w386:refnum<class "Inst UI.AH2500.lvclass">, "Instrument"=w385:refnum<class "Inst.AH2500.lvclass">)
            n131 = call <vilib>:"GetProtectedEvents.vi"("SMO"=w386) -> ("error out"=w389:errorcluster, "SMO Protected Events"=w391:T12)  [unwired: 8 in, 1 out]
            n132 = call <userlib>:"Instrument.GetPublicEvents.vi"("Instrument"=w385) -> ("error out"=w387:errorcluster, "Instrument Public Events"=w388:T13, "Instrument out"=w383:refnum<class "Inst.AH2500.lvclass">)  [unwired: 8 in]
            n133 = call "Inst.AH2500.GetPublicEvents.vi"("Inst.AH2500 in"=w383) -> ("error out"=w382:errorcluster, "Inst.AH2500 Public Events"=w384:T14, "Inst.AH2500 out"=w379:refnum<class "Inst.AH2500.lvclass">)  [unwired: 8 in]
            n134 = call <vilib>:"GetPublicEvents.vi"("SMO"=w379) -> ("error out"=w377:errorcluster, "Public Events"=w378:T15)  [unwired: 8 in, 1 out]
            n135 = register-events(w391, w388, w384, w378) -> (reference out=w392:refnum<event-registration>, error out=w381:errorcluster)  [unwired: 2 in]
            n136 = Merge Errors(w381, w377, w382, w387, w389, w380) -> (w390:errorcluster)
            n137 = call <vilib>:"Add State(s) to Queue__jki_lib_state_machine.vi"("State(s) in (\"\")"=w395) -> ("States Out"=w394:string)  [unwired: 14 in]
          }
          frame "Events: Unregister" {
            n138 = Unregister For Events(event registration refnum=w398, error in=w397) -> (error out=w396:errorcluster)
            n139 = call <vilib>:"Add State(s) to Queue__jki_lib_state_machine.vi"("State(s) in (\"\")"=w401) -> ("States Out"=w400:string)  [unwired: 14 in]
          }
          frame "---------- Configuration ----------" {
            # "Do not put any code in this frame.\n(It is a separator no-op. You can make a copy of this frame to create a new UI frame)"
            n140 = call <vilib>:"Add State(s) to Queue__jki_lib_state_machine.vi"("State(s) in (\"\")"=w406) -> ("States Out"=w405:string)  [unwired: 14 in]
          }
          frame "Configuration: Initialize" {
            # "Do not put any code in this frame.\n(It is a separator no-op. You can make a copy of this frame to create a new UI frame)"
            n141 = Unbundle By Name(w414) -> ("Configuration"=w412:refnum<class "Configuration.lvclass">, "Instrument"=w413:refnum<class "Inst.AH2500.lvclass">)
            n142 = call <vilib>:"GetName.vi"("error in (no error)"=w416, "SMO"=w413) -> ("error out"=w415:errorcluster, "Name"=w417:string)  [unwired: 6 in, 2 out]
            n143 = call <userlib>:"Default Path.vi"("error in (no error)"=w415, "Folder Name [Application Name]"=w417, "Configuration in"=w412) -> ("error out"=w408:errorcluster, "Configuration out"=w411:refnum<class "Configuration.lvclass">)  [unwired: 7 in]
            n144 = call <userlib>:"Write Section.vi"("error in (no error)"=w408, "Section"="UI", "Configuration in"=w411) -> ("error out"=w407:errorcluster, "Configuration out"=w410:refnum<class "Configuration.lvclass">)  [unwired: 7 in]
            n145 = Bundle By Name(cluster=w414, "Configuration"=w410) -> (w418:T9)
            n146 = call <vilib>:"Add State(s) to Queue__jki_lib_state_machine.vi"("State(s) in (\"\")"=w421) -> ("States Out"=w420:string)  [unwired: 14 in]
          }
          frame "Configuration: Write UI Config File" {
            # "Do not put any code in this frame.\n(It is a separator no-op. You can make a copy of this frame to create a new Data frame)"
            n147 = Unbundle By Name(w426) -> ("Configuration"=w423:refnum<class "Configuration.lvclass">, "UI Cluster"=w425:T7)
            n148 = call <userlib>:"Write Configuration.vi"("error in (no error)"=w422, "Variant"=w425, "Configuration in"=w423) -> ("error out"=w424:errorcluster)  [unwired: 7 in, 1 out]
            n149 = call <vilib>:"Add State(s) to Queue__jki_lib_state_machine.vi"("State(s) in (\"\")"=w429) -> ("States Out"=w428:string)  [unwired: 14 in]
          }
          frame "Configuration: Read UI Config File" {
            # "Do not put any code in this frame.\n(It is a separator no-op. You can make a copy of this frame to create a new UI frame)"
            n150 = Unbundle By Name(w432) -> ("UI Cluster"=w435:T7, "Configuration"=w438:refnum<class "Configuration.lvclass">)
            n151 = call <userlib>:"Read Configuration.vi"("INI Fomatted Cluster Type"=w435, "error in (no error)"=w434, "Configuration in"=w438) -> ("error out"=w437:errorcluster, "Configuration"=w436:variant)  [unwired: 6 in, 1 out]
            n152 = Variant To Data(error in=w437, type=w435, Variant=w436) -> (data=w431:T7, error out=w433:errorcluster)
            n153 = Bundle By Name(cluster=w432, "UI Cluster"=w431) -> (w430:T9)
            n154 = call <vilib>:"Add State(s) to Queue__jki_lib_state_machine.vi"("State(s) in (\"\")"=w441) -> ("States Out"=w440:string)  [unwired: 14 in]
          }
          frame "---------- Action ----------" {
            n155 = Unbundle By Name(w443) -> ("Instrument"=w444:refnum<class "Inst.AH2500.lvclass">)
            n156 = Bundle By Name(cluster=w443, "Instrument"=w444) -> (w442:T9)
            n157 = call <vilib>:"Add State(s) to Queue__jki_lib_state_machine.vi"("State(s) in (\"\")"=w448) -> ("States Out"=w447:string)  [unwired: 14 in]
          }
          frame "Action: Notify UI Closed" {
            # "Notify that the UI has been closed"
            n158 = Unbundle By Name(w449) -> ("Instrument UI"=w452:refnum<class "Inst UI.AH2500.lvclass">)
            n159 = call <vilib>:"Hide.vi"("error in (no error)"=w451, "SMO.UI"=w452) -> ("error out"=w450:errorcluster)  [unwired: 8 in, 1 out]
            n160 = call <vilib>:"Add State(s) to Queue__jki_lib_state_machine.vi"("State(s) in (\"\")"=w455) -> ("States Out"=w454:string)  [unwired: 14 in]
          }
          frame "Action: getAll" {
            n161 = Unbundle By Name(w462) -> ("getAll"=w460:T6, "Instrument"=w465:refnum<class "Inst.AH2500.lvclass">)
            n162 = call <userlib>:"getAll.vi"("error in (no error)"=w463, "Instrument in"=w465) -> ("error out"=w456:errorcluster, "getAll"=w459:variant, "Instrument out"=w461:refnum<class "Inst.AH2500.lvclass">)  [unwired: 7 in]
            n163 = call "JSON to LVtype.vim"("type"=w460, "error in (no error)"=w456, "JSON Data in"=w459) -> ("error out"=w457:errorcluster, "Data out"=w458:T6)  [unwired: 7 in]
            n164 = Bundle By Name(cluster=w462, "Instrument"=w461, "getAll"=w458) -> (w464:T9)
            n165 = call <vilib>:"Add State(s) to Queue__jki_lib_state_machine.vi"("State(s) in Front (\"\")"="" ("State(s) in Front (\"\")"), "State(s) in (\"\")"=w469) -> ("States Out"=w468:string)  [unwired: 13 in]
          }
          frame "Action: Open" {
            n166 = Unbundle By Name(w475) -> ("Instrument"=w474:refnum<class "Inst.AH2500.lvclass">)
            n167 = call <userlib>:"Write Client Type.vi"("error in (no error)"=w471, "Client Type [Remote]"=Client_Type--Enum."Local" ("Client Type"), "Instrument in"=w474) -> ("error out"=w472:errorcluster, "Instrument out"=w473:refnum<class "Inst.AH2500.lvclass">)  [unwired: 7 in]
            n168 = Bundle By Name(cluster=w475, "Instrument"=w473) -> (w476:T9)
            n169 = call <vilib>:"Add State(s) to Queue__jki_lib_state_machine.vi"("State(s) in Front (\"\")"="" ("State(s) in Front (\"\")"), "State(s) in (\"\")"=w480) -> ("States Out"=w479:string)  [unwired: 13 in]
          }
          frame "Action: Close" {
            n170 = Unbundle By Name(w481) -> ("Instrument"=w484:refnum<class "Inst.AH2500.lvclass">)
            n171 = Bundle By Name(cluster=w481, "Instrument"=w484) -> (w483:T9)
            n172 = call <vilib>:"Add State(s) to Queue__jki_lib_state_machine.vi"("State(s) in Front (\"\")"="" ("State(s) in Front (\"\")"), "State(s) in (\"\")"=w488) -> ("States Out"=w487:string)  [unwired: 13 in]
          }
          frame "Action: Send Message to Instrument" {
            # "Send a message (command, data, etc) to the Instrument:process.vi"
            n173 = Unbundle By Name(w493) -> ("Instrument"=w492:refnum<class "Inst.AH2500.lvclass">)  [unwired: 1 out]
            n174 = call-poly <userlib>:"Instrument.sendMessageToProcess.vi"("error in (no error)"=w490, "Instrument"=w492) -> ("error out"=w489:errorcluster, "Instrument out"=w491:refnum<class "Inst.AH2500.lvclass">)  [unwired: 8 in]
            n175 = Bundle By Name(cluster=w493, "Instrument"=w491) -> (w494:T9)
            n176 = call <vilib>:"Add State(s) to Queue__jki_lib_state_machine.vi"("State(s) in Front (\"\")"="" ("State(s) in Front (\"\")"), "State(s) in (\"\")"=w498) -> ("States Out"=w497:string)  [unwired: 13 in]
          }
          frame "Action: Send Message to Child" {
            # "Send a message (command, data, etc) to the Instrument.Child:process.vi"
            n177 = Unbundle By Name(w503) -> ("Instrument"=w502:refnum<class "Inst.AH2500.lvclass">)  [unwired: 1 out]
            n178 = call "Inst.AH2500.MessageToProcess.vi"("error in (no error)"=w500, "Inst.AH2500 in"=w502) -> ("error out"=w499:errorcluster, "Inst.AH2500 out"=w501:refnum<class "Inst.AH2500.lvclass">)  [unwired: 8 in]
            n179 = Bundle By Name(cluster=w503, "Instrument"=w501) -> (w504:T9)
            n180 = call <vilib>:"Add State(s) to Queue__jki_lib_state_machine.vi"("State(s) in Front (\"\")"="" ("State(s) in Front (\"\")"), "State(s) in (\"\")"=w508) -> ("States Out"=w507:string)  [unwired: 13 in]
          }
        }
      }
    }
    frame Error {
    }
  }
  n181 = call-parent "Process.vi"("error in"=w5, "Instrument UI in"=w4) -> ("error out"=w2:errorcluster, "Instrument UI out"=→"Inst UI.AH2500 out":refnum<class "Inst UI.AH2500.lvclass">)  [unwired: 8 in]
  n182 = Merge Errors(w2, w1) -> (→"error out":errorcluster)
